vi "Take_photo.vi"(7 "error in":errorcluster, 10 "Session In":T2) -> (0 "error out":errorcluster, 2 "x = y?":bool)   [LabVIEW 2020]
doc: "Take photo if matching template."
uses:
  <vilib>/userDefined/High Color/IMAQdx.ctl
  <vilib>/vision/driver/NI_Vision_Acquisition_Software.lvlib
  <vilib>/vision/NI_Vision_Development_Module.lvlib
panel:
  out "Application Directory 3":path
  out "Application Directory 2":path
  out "Number of Matches":i32
  out "Image 2":T1(plugin-control)
  out "Image":T1(plugin-control)
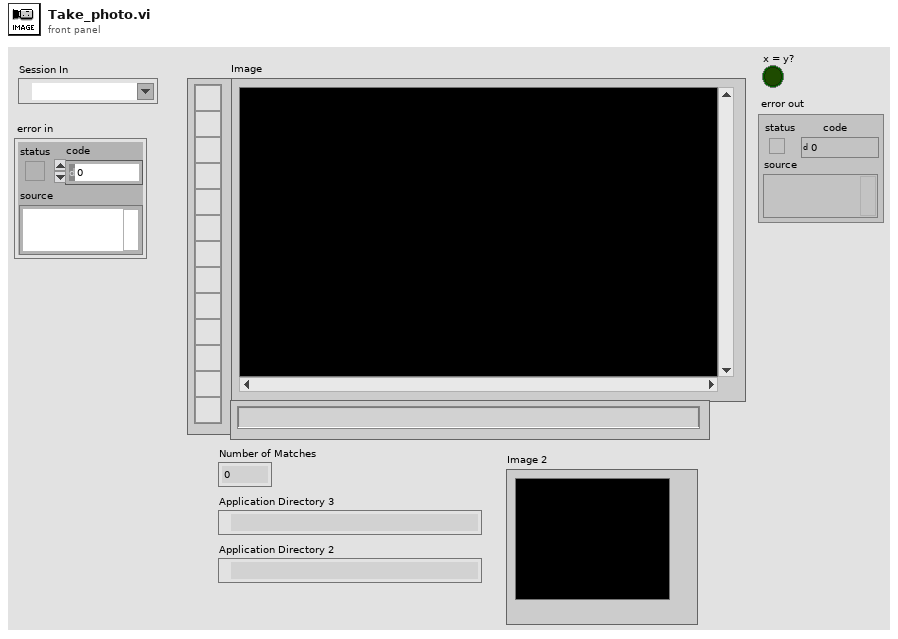
[diagram p1: front panel]
types:
  T1 = typedef "IMAQ Image.ctl" = refnum<image>
  T2 = typedef "IMAQdx.ctl" = refnum<k21>
  T3 = cluster{"Position":cluster{"x":sgl, "y":sgl}, "Angle":sgl, "Scale":sgl, "Score":sgl, "Bounding Box":cluster{"x":sgl, "y":sgl}[]}[]
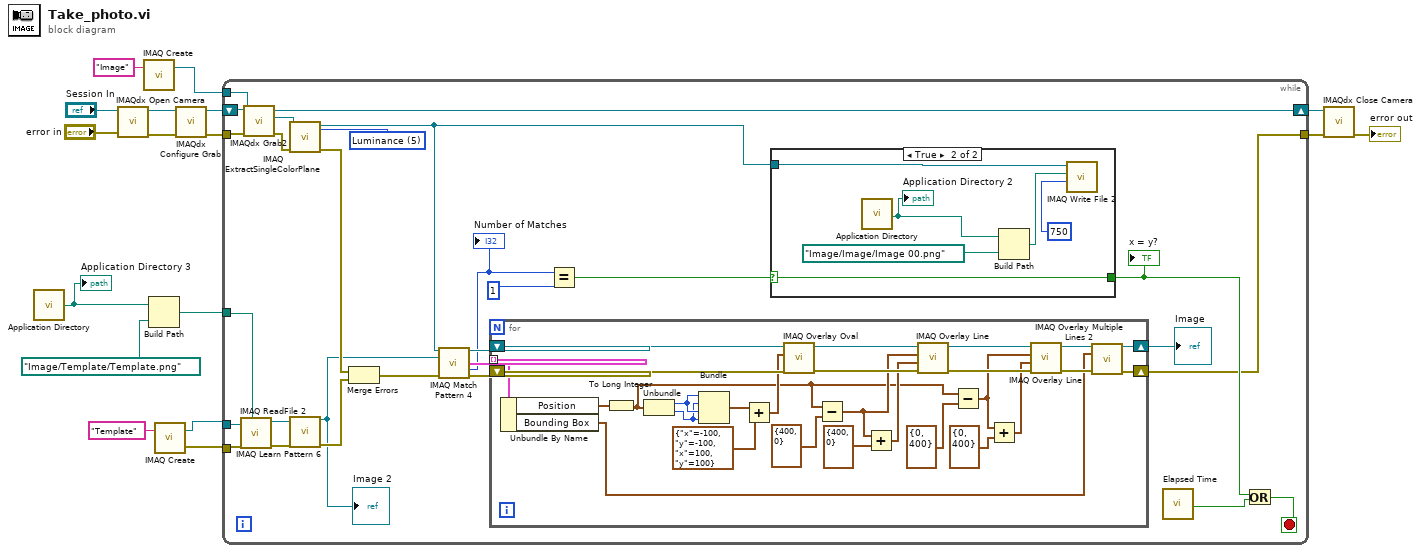
[diagram p0: block diagram]
diagram:
  n1 = call <vilib>:"Application Directory.vi"() -> ("Application Directory"=w4:path)
  "Application Directory 3" <- w4
  n2 = call <vilib>:"IMAQdx Open Camera.vi"("error in"="error in", "Session In"="Session In") -> ("error out"=w16:errorcluster, "Session Out"=w15:T2)  [unwired: 8 in]
  n3 = call "IMAQ Create"("Image Name"="Image") -> ("New Image"=w10:T1)  [unwired: 4 in, 1 out]
  n4 = Build Path(base path=w4, name or relative path=path "Image/Template/Template.png") -> (appended path=w6:path)
  n5 = call "IMAQ Create"("Image Name"="Template") -> ("New Image"=w8:T1, "error out"=w7:errorcluster)  [unwired: 4 in]
  n6 = call <vilib>:"IMAQdx Configure Grab.vi"("error in"=w16, "Session In"=w15) -> ("error out"=w12:errorcluster, "Session Out"=w13:T2)  [unwired: 8 in]
  n7 = while {
    tunnel: w12 -> [w45]
    shift-right: [w44] -> w11
    shift-left: w13 -> [w42]
    tunnel: w10 -> [w43]
    tunnel: w8 -> [w39]
    tunnel: w6 -> [w30]
    tunnel: w7 -> [w28]
    tunnel: [w20] -> w2
    stop <- w24 stop-if-true
    w41 = 5 items=["Red", "Green", "Blue", "Hue", "Saturation", "Luminance", "Value", "Intensity"] ("Color Plane")
    n8 = call "IMAQ ReadFile 2"("File Path"=w30, "error in (no error)"=w28, "Image"=w39) -> ("error out"=w37:errorcluster, "Image Out"=w38:T1)  [unwired: 4 in, 3 out]
    n9 = call <vilib>:"IMAQdx Grab2.vi"("error in"=w45, "Image In"=w43, "Session In"=w42) -> ("error out"=w29:errorcluster, "Image Out"=w40:T1, "Session Out"=w44:T2)  [unwired: 5 in, 1 out]
    n10 = call "IMAQ ExtractSingleColorPlane"("Color Plane"=w41, "error in (no error)"=w29, "Image Src"=w40) -> ("error out"=w23:errorcluster, "Image Dst Out"=w36:T1)  [unwired: 1 in, 6 out]
    n11 = call "IMAQ Learn Pattern 6"("Image"=w38, "error in (no error)"=w37) -> ("Template Image Out"=w19:T1, "error out"=w22:errorcluster)  [unwired: 11 in, 1 out]
    "Image 2" <- w19
    n12 = Merge Errors(w23, w22) -> (w21:errorcluster)
    n13 = call "IMAQ Match Pattern 4"("Image"=w36, "Template Image"=w19, "error in (no error)"=w21) -> ("Image (duplicate)"=w35:T1, "Matches (real-world)"=w33:T3, "Number of Matches"=w32:i32, "error out"=w34:errorcluster)  [unwired: 8 in, 1 out]
    "Number of Matches" <- w32
    n14 = for {
      tunnel: w33 -> [w63] mode=indexing
      shift-right: [w68] -> w18
      shift-left: w35 -> [w72]
      shift-right: [w47] -> w20
      shift-left: w34 -> [w67]
      n15 = Unbundle By Name(w63) -> ("Position"=w55:cluster{"x":sgl, "y":sgl}, "Bounding Box"=w46:cluster{"x":sgl, "y":sgl}[])
      n16 = To Long Integer(number=w55) -> (32bit integer=w54:cluster{"x":i32, "y":i32})
      n17 = Unbundle(w54) -> ("x"=w62:i32, "y"=w61:i32)
      n18 = Bundle("x"=w62, "y"=w61, "x"=w62, "y"=w61) -> (w60:cluster{"x":i32, "y":i32, "x":i32, "y":i32})  [unwired: 1 in]
      n19 = Add(x=w60, y=cluster{"x":i32, "y":i32, "x":i32, "y":i32} {"x"=-100, "y"=-100, "x"=100, "y"=100}) -> (x+y=w59:cluster{"x":i32, "y":i32, "x":i32, "y":i32})
      n20 = call "IMAQ Overlay Oval"("error in (no error)"=w67, "Bounding Rectangle"=w59, "Image"=w72) -> ("error out"=w66:errorcluster, "Image Out"=w71:T1)  [unwired: 7 in]
      n21 = Subtract(x=w54, y=cluster{"x":i32, "y":i32} {"x"=400, "y"=0}) -> (x-y=w57:cluster{"x":i32, "y":i32})
      n22 = Add(x=w57, y=cluster{"x":i32, "y":i32} {"x"=400, "y"=0}) -> (x+y=w56:cluster{"x":i32, "y":i32})
      n23 = call "IMAQ Overlay Line"("error in (no error)"=w66, "End Point"=w56, "Start Point"=w57, "Image"=w71) -> ("error out"=w65:errorcluster, "Image Out"=w70:T1)  [unwired: 6 in]
      n24 = Subtract(x=w54, y=cluster{"x":i32, "y":i32} {"x"=0, "y"=400}) -> (x-y=w50:cluster{"x":i32, "y":i32})
      n25 = Add(x=w50, y=cluster{"x":i32, "y":i32} {"x"=0, "y"=400}) -> (x+y=w48:cluster{"x":i32, "y":i32})
      n26 = call "IMAQ Overlay Line"("error in (no error)"=w65, "End Point"=w48, "Start Point"=w50, "Image"=w70) -> ("error out"=w64:errorcluster, "Image Out"=w69:T1)  [unwired: 6 in]
      n27 = call "IMAQ Overlay Multiple Lines 2"("Image"=w69, "Line End Points"=w46, "error in (no error)"=w64) -> ("Image Out"=w68:T1, "error out"=w47:errorcluster)  [unwired: 11 in]
    }
    "Image" <- w18
    n28 = Equal?(x=w32, y=1) -> (x = y?=w27:bool)
    n29 = case shown="True" w27 {
      selector: w27 -> [w73 w77]
      tunnel: w36 -> [_ w78]
      tunnel: [w73 w77] -> w25
      frame False {
      }
      frame True {
        n30 = call <vilib>:"Application Directory.vi"() -> ("Application Directory"=w74:path)
        "Application Directory 2" <- w74
        n31 = Build Path(base path=w74, name or relative path=path "Image/Image/Image 00.png") -> (appended path=w76:path)
        n32 = call-poly "IMAQ Write File 2"("Image Quality"=u32 750, "File Path"=w76, "Image"=w78) -> ()  [unwired: 7 in, 2 out]
      }
    }
    "x = y?" <- w25
    n33 = call "Elapsed Time"() -> ("Time has Elapsed"=w26:bool)  [unwired: 12 in, 7 out]
    n34 = Or(x=w26, y=w25) -> (x .or. y?=w24:bool)
  }
  n35 = call <vilib>:"IMAQdx Close Camera.vi"("error in"=w2, "Session In"=w11) -> ("error out"=→"error out":errorcluster)  [unwired: 9 in]
